vi "MH_AllDllFunctions_AnyThread.vi"   [LabVIEW 2017]
uses:
  mhlib_x86_x64_AnyThread.llb/MH_DllPath_global.vi
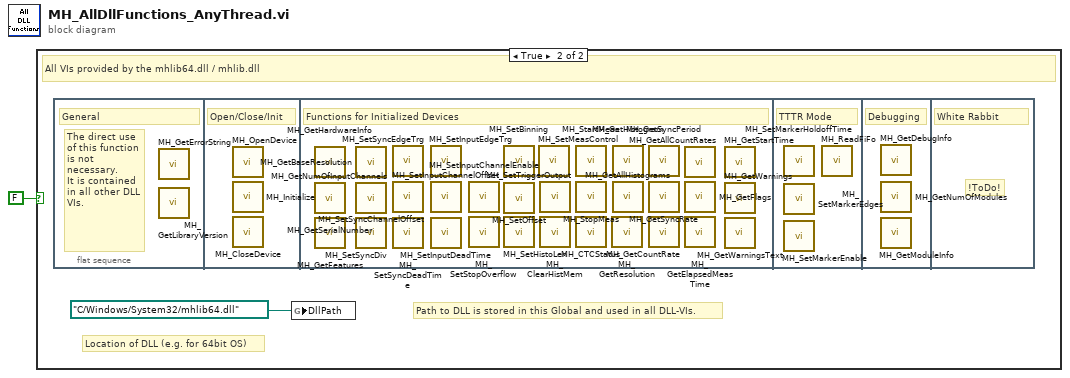
[diagram p0: block diagram]
diagram:
  n1 = case shown="True" FALSE {
    frame False {
    }
    frame True {
      # "Location of DLL (e.g. for 64bit OS)"
      # "Path to DLL is stored in this Global and used in all DLL-VIs."
      # "All VIs provided by the mhlib64.dll / mhlib.dll"
      n2 = flat-sequence {
        frame #0 {
          # "The direct use of this function is not necessary.\nIt is contained in all other DLL VIs."
          # "General"
          n3 = call "MH_GetErrorString.vi"() -> ()  [unwired: 9 in, 3 out]
          n4 = call "MH_GetLibraryVersion.vi"() -> ()  [unwired: 9 in, 3 out]
        }
        frame #1 {
          # "Open/Close/Init"
          n5 = call "MH_OpenDevice.vi"() -> ()  [unwired: 9 in, 3 out]
          n6 = call "MH_Initialize.vi"() -> ()  [unwired: 10 in, 2 out]
          n7 = call "MH_CloseDevice.vi"() -> ()  [unwired: 10 in, 2 out]
        }
        frame #2 {
          # "Functions for Initialized Devices"
          n8 = call "MH_GetHardwareInfo.vi"() -> ()  [unwired: 7 in, 5 out]
          n9 = call "MH_GetSerialNumber.vi"() -> ()  [unwired: 9 in, 3 out]
          n10 = call "MH_GetFeatures.vi"() -> ()  [unwired: 9 in, 3 out]
          n11 = call "MH_GetBaseResolution.vi"() -> ()  [unwired: 8 in, 4 out]
          n12 = call "MH_GetNumOfInputChannels.vi"() -> ()  [unwired: 9 in, 3 out]
          n13 = call "MH_SetSyncDiv.vi"() -> ()  [unwired: 10 in, 2 out]
          n14 = call "MH_SetSyncEdgeTrg.vi"() -> ()  [unwired: 10 in, 2 out]
          n15 = call "MH_SetSyncChannelOffset.vi"() -> ()  [unwired: 10 in, 2 out]
          n16 = call "MH_SetSyncDeadTime.vi"() -> ()  [unwired: 10 in, 2 out]
          n17 = call "MH_SetInputEdgeTrg.vi"() -> ()  [unwired: 10 in, 2 out]
          n18 = call "MH_SetInputChannelOffset.vi"() -> ()  [unwired: 10 in, 2 out]
          n19 = call "MH_SetInputDeadTime.vi"() -> ()  [unwired: 10 in, 2 out]
          n20 = call "MH_SetInputChannelEnable.vi"() -> ()  [unwired: 10 in, 2 out]
          n21 = call "MH_SetStopOverflow.vi"() -> ()  [unwired: 10 in, 2 out]
          n22 = call "MH_SetBinning.vi"() -> ()  [unwired: 10 in, 2 out]
          n23 = call "MH_SetOffset.vi"() -> ()  [unwired: 10 in, 2 out]
          n24 = call "MH_SetHistoLen.vi"() -> ()  [unwired: 9 in, 3 out]
          n25 = call "MH_SetMeasControl.vi"() -> ()  [unwired: 10 in, 2 out]
          n26 = call "MH_SetTriggerOutput.vi"() -> ()  [unwired: 10 in, 2 out]
          n27 = call "MH_ClearHistMem.vi"() -> ()  [unwired: 10 in, 2 out]
          n28 = call "MH_StartMeas.vi"() -> ()  [unwired: 10 in, 2 out]
          n29 = call "MH_StopMeas.vi"() -> ()  [unwired: 10 in, 2 out]
          n30 = call "MH_CTCStatus.vi"() -> ()  [unwired: 9 in, 3 out]
          n31 = call "MH_GetResolution.vi"() -> ()  [unwired: 9 in, 3 out]
          n32 = call "MH_GetHistogram.vi"() -> ()  [unwired: 9 in, 3 out]
          n33 = call "MH_GetAllHistograms.vi"() -> ()  [unwired: 9 in, 3 out]
          n34 = call "MH_GetSyncPeriod.vi"() -> ()  [unwired: 9 in, 3 out]
          n35 = call "MH_GetSyncRate.vi"() -> ()  [unwired: 9 in, 3 out]
          n36 = call "MH_GetCountRate.vi"() -> ()  [unwired: 9 in, 3 out]
          n37 = call "MH_GetAllCountRates.vi"() -> ()  [unwired: 8 in, 4 out]
          n38 = call "MH_GetFlags.vi"() -> ()  [unwired: 9 in, 3 out]
          n39 = call "MH_GetElapsedMeasTime.vi"() -> ()  [unwired: 9 in, 3 out]
          n40 = call "MH_GetStartTime.vi"() -> ()  [unwired: 7 in, 5 out]
          n41 = call "MH_GetWarnings.vi"() -> ()  [unwired: 9 in, 3 out]
          n42 = call "MH_GetWarningsText.vi"() -> ()  [unwired: 9 in, 3 out]
        }
        frame #3 {
          # "TTTR Mode"
          n43 = call "MH_SetMarkerHoldoffTime.vi"() -> ()  [unwired: 10 in, 2 out]
          n44 = call "MH_SetMarkerEdges.vi"() -> ()  [unwired: 10 in, 2 out]
          n45 = call "MH_SetMarkerEnable.vi"() -> ()  [unwired: 10 in, 2 out]
          n46 = call "MH_ReadFiFo.vi"() -> ()  [unwired: 8 in, 4 out]
        }
        frame #4 {
          # "Debugging"
          n47 = call "MH_GetDebugInfo.vi"() -> ()  [unwired: 9 in, 3 out]
          n48 = call "MH_GetNumOfModules.vi"() -> ()  [unwired: 9 in, 3 out]
          n49 = call "MH_GetModuleInfo.vi"() -> ()  [unwired: 8 in, 4 out]
        }
        frame #5 {
          # "!ToDo!"
          # "White Rabbit"
        }
      }
      n50 = global write "MH_DllPath_global.vi" "DllPath"(path "C:/Windows/System32/mhlib64.dll" ("DllPath")) -> ()
    }
  }
